vi "mailRapportExped.vi"(0 "chaine valves":string="12-216C-04521 EQIFIL 417mA 14.4ohm\t112105740008030109\t18.04.2008 15:35\tMQI\t12345/06-03.03.03\t2\t30\r\n12-216C-04521 EQIFIL 417mA 14.4ohm\t112105740008030108\t18.04.2008 15:35\tMQI\t12345/06-03.03.03\t2\t30\r\n12-216C-04521 EQIFIL 417mA 14.4ohm\t112105740008030107\t18.04.2008 15:35\tMQI\t12345/06-03.03.03\t2\t30\r\n12-216C-04521 EQIFIL 417mA 14.4ohm\t112105740008030106\t18.04.2008 15:35\tMQI\t12345/06-03.03.03\t2\t30\r\n12-216C-04521 EQIFIL 417mA 14.4ohm\t112105740008030105\t18.04.2008 15:35\tMQI\t12345/06-03.03.03\t2\t30\r\n12-216C-04521 EQIFIL 417mA 14.4ohm\t112105740008030104\t18.04.2008 15:35\tMQI\t12345/06-03.03.03\t1\t30\r\n12-216C-04521 EQIFIL 417mA 14.4ohm\t112105740008030103\t18.04.2008 15:34\tMQI\t12345/06-03.03.03\t1\t30\r\n12-216C-04521 EQIFIL 417mA 14.4ohm\t112105740008030102\t18.04.2008 15:34\tMQI\t12345/06-03.03.03\t1\t30\r\n12-216C-04521 EQIFIL 417mA 14.4ohm\t112105740008030101\t18.04.2008 15:34\tMQI\t12345/06-03.03.03\t1\t30\r\n12-216C-04521 EQIFIL 417mA 14.4ohm\t112105740008030100\t18.04.2008 15:34\tMQI\t12345/06-03.03.03\t1\t30\r\n12-216C-04521 EQIFIL 417mA 14.4ohm\t112105740008020106\t18.04.2008 15:34\tMQI\t12345/06-03.03.03\t1\t30\r\n12-216C-04521 EQIFIL 417mA 14.4ohm\t112105740008020105\t18.04.2008 15:34\tMQI\t12345/06-03.03.03\t1\t30\r\n12-216C-04521 EQIFIL 417mA 14.4ohm\t112105740008020104\t18.04.2008 15:34\tMQI\t12345/06-03.03.03\t1\t30\r\n12-216C-04521 EQIFIL 417mA 14.4ohm\t112105740008020103\t18.04.2008 15:34\tMQI\t12345/06-03.03.03\t1\t30\r\n12-216C-04521 EQIFIL 417mA 14.4ohm\t112105740008020102\t18.04.2008 15:34\tMQI\t12345/06-03.03.03\t1\t30\r\n12-216C-04521 EQIFIL 417mA 14.4ohm\t112105740008020101\t18.04.2008 15:34\tMQI\t12345/06-03.03.03\t1\t30\r\n12-216C-04521 EQIFIL 417mA 14.4ohm\t112105740008020100\t18.04.2008 15:34\tMQI\t12345/06-03.03.03\t1\t30\r\n12-216C-04521 EQIFIL 417mA 14.4ohm\t112105740008010112\t18.04.2008 15:34\tMQI\t12345/06-03.03.03\t1\t30\r\n12-216C-04521 EQIFIL 417mA 14.4ohm\t112105740008010111\t18.04.2008 15:34\tMQI\t12345/06-03.03.03\t1\t30\r\n12-216C-04521 EQIFIL 417mA 14.4ohm\t112105740008010110\t18.04.2008 15:34\tMQI\t12345/06-03.03.03\t1\t30\r\n12-216C-04521 EQIFIL 417mA 14.4ohm\t112105740008010109\t18.04.2008 15:34\tMQI\t12345/06-03.03.03\t1\t30\r\n12-216C-04521 EQIFIL 417mA 14.4ohm\t112105740008010108\t18.04.2008 15:34\tMQI\t12345/06-03.03.03\t1\t30\r\n12-216C-04521 EQIFIL 417mA 14.4ohm\t112105740008010107\t18.04.2008 15:34\tMQI\t12345/06-03.03.03\t1\t30\r\n12-216C-04521 EQIFIL 417mA 14.4ohm\t112105740008010106\t18.04.2008 15:34\tMQI\t12345/06-03.03.03\t1\t30\r\n12-216C-04521 EQIFIL 417mA 14.4ohm\t112105740008010105\t18.04.2008 15:34\tMQI\t12345/06-03.03.03\t1\t30\r\n12-216C-04521 EQIFIL 417mA 14.4ohm\t112105740008010104\t18.04.2008 15:34\tMQI\t12345/06-03.03.03\t1\t30\r\n12-216C-04521 EQIFIL 417mA 14.4ohm\t112105740008010103\t18.04.2008 15:33\tMQI\t12345/06-03.03.03\t1\t30\r\n12-216C-04521 EQIFIL 417mA 14.4ohm\t112105740008010102\t18.04.2008 15:33\tMQI\t12345/06-03.03.03\t1\t30\r\n12-216C-04521 EQIFIL 417mA 14.4ohm\t112105740008010101\t18.04.2008 15:33\tMQI\t12345/06-03.03.03\t1\t30\r\n12-216C-04521 EQIFIL 417mA 14.4ohm\t112105740008010100\t18.04.2008 15:33\tMQI\t12345/06-03.03.03\t1\t30\r\n", 3 "produit":string, 5 "DATA cmde":T1, 7 "chemin de base":path, 9 "Email Expédition":string="marion.quiquerez@fas.ch", 11 "error in (no error)":errorcluster caption="entrée d'erreur (pas d'erreur)", 12 "n° cmde":string, 14 "tab histo filtré\n par n° cmde":string[][](array[string])) -> (4 "Texte fichier":string, 6 "Titre fichier":string, 15 "error out":errorcluster caption="sortie d'erreur")   [LabVIEW 2020]
doc: "Envoi un mail avec la liste des valves emballées en pièce jointe si spécifié dans le fichier XML PP de la valve (FlatProp) ou correspondance produit code barre.txt (autres valves)"
uses:
  <vilib>/Utility/SMTP/NI_SMTPEmail.lvlib
panel:
  out "valeur max":string
  out "Texte mail":string caption="Résultat"
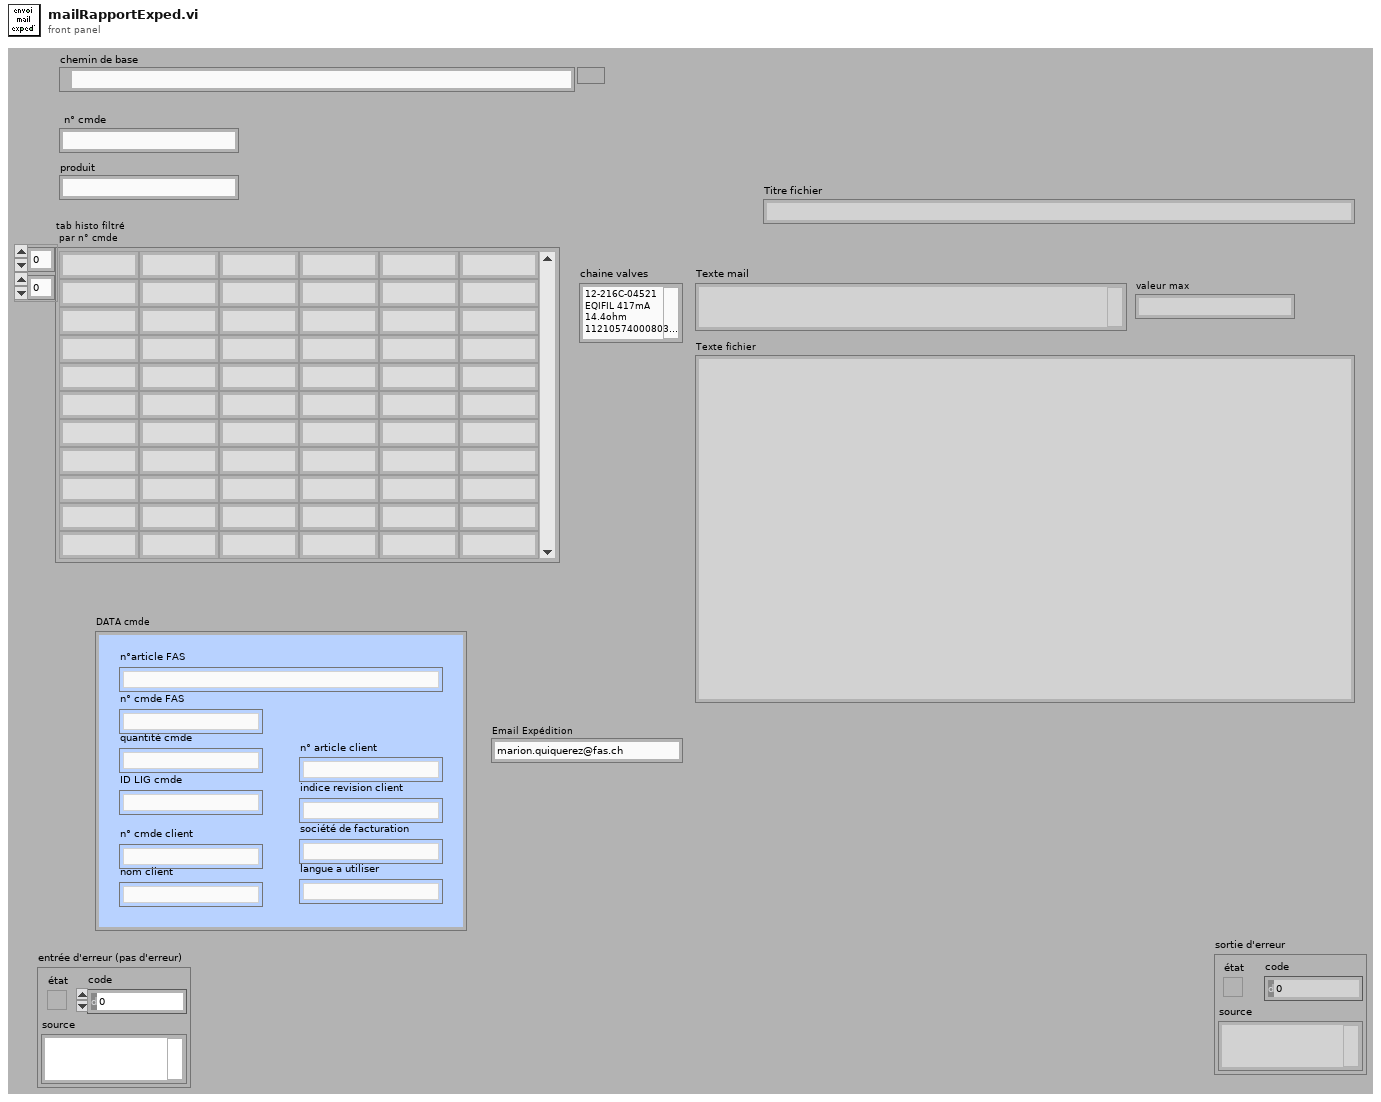
[diagram p1: front panel]
types:
  T1 = typedef "DATA commande.ctl" = cluster{"n°article FAS":string, "n° cmde FAS":string, "quantité cmde":string, "ID LIG cmde":string, "n° cmde client":string, "nom client":string, "n° article client":string, "indice revision client":string, "société de facturation":string, "langue a utiliser":string}
  T2 = enum16{"open", "replace", "create", "open or create", "replace or create", "replace or create with confirmation"}
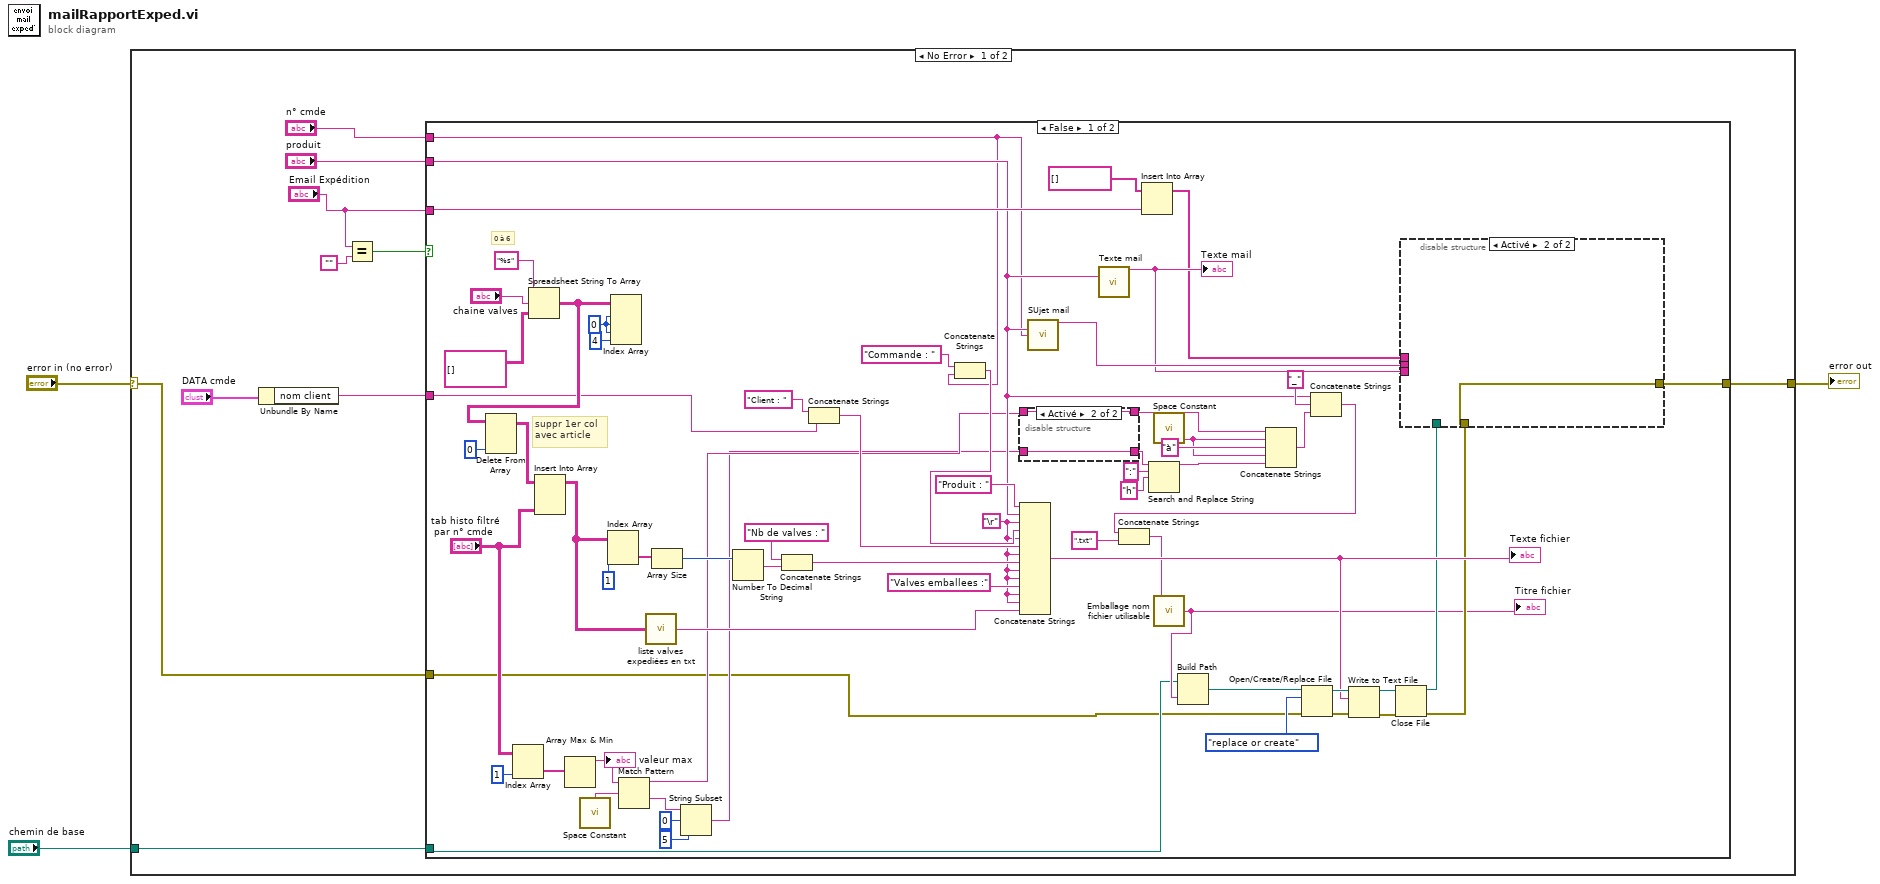
[diagram p0: block diagram]
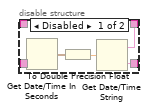
[diagram p2: hidden frame]
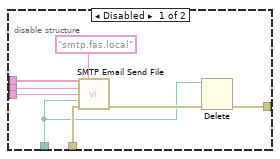
[diagram p3: hidden frame]
diagram:
  n1 = case shown="No Error" "error in (no error)" {
    selector: "error in (no error)" -> [w12 w96]
    tunnel: [w13 w96] -> w3
    tunnel: "chemin de base" -> [w4 _]
    frame No Error {
      n2 = Unbundle By Name("DATA cmde") -> ("nom client"=w7:string)
      n3 = Equal?(x="Email Expédition", y="") -> (x = y?=w9:bool)
      n4 = case shown="False" w9 {
        tunnel: [w53 w95] -> w13
        tunnel: w12 -> [w14 w95]
        tunnel: "Email Expédition" -> [w30 _]
        tunnel: w7 -> [w32 _]
        tunnel: "produit" -> [w27 _]
        tunnel: "n° cmde" -> [w26 _]
        tunnel: w4 -> [w15 _]
        frame False {
          w62 = 0 ("indice désactivé (col)")
          w49 = "\r"
          # "suppr 1er col \navec article"
          # "0 à 6"
          n5 = Index Array(array="tab histo filtré\n par n° cmde", index (col)=1 ("indice désactivé (col)")) -> (element=w23:string[])  [unwired: 1 in]
          n6 = Spreadsheet String To Array(format string="%s" ("chaîne de format"), spreadsheet string="chaine valves", array type (2D Dbl)=string[][] [] ("type de tableau (2D de dbl)")) -> (array=w36:string[][])  [unwired: 1 in]
          n7 = Delete From Array(array=w36, index (col)=0 ("indice désactivé (col)")) -> (array with subset deleted=w34:string[][])  [unwired: 2 in, 1 out]
          n8 = Insert Into Array(array=w34, new element="tab histo filtré\n par n° cmde") -> (w31:string[][])  [unwired: 2 in]
          n9 = Array Max & Min(array=w23) -> (max value=w22:string)  [unwired: 3 out]
          "valeur max" <- w22
          n10 = call <vilib>:"Space Constant.vi"() -> ("String"=w21:string)
          n11 = Index Array(array=w31, index (col)=1 ("indice désactivé (col)")) -> (element=w58:string[])  [unwired: 1 in]
          n12 = Index Array(array=w36, index (row) #1=w62, index (col) #1=w62, index (row) #2=w62, index (col) #2=4 ("indice désactivé (col)")) -> ()  [unwired: 2 out]
          n13 = Match Pattern(string=w22, regular expression=w21) -> (before substring=w20:string, after substring=w19:string)  [unwired: 1 in, 2 out]
          n14 = call "liste valves expediées en txt.vi"("Tab valves"=w31) -> ("liste valves"=w50:string)
          n15 = Array Size(array=w58) -> (size(s)=w33:i32)
          n16 = String Subset(string=w19, offset (0)=0, length (rest)=5 ("longueur (reste)")) -> (substring=w16:string)
          n17 = Number To Decimal String(number=w33) -> (decimal integer string=w56:string)  [unwired: 1 in]
          n18 = Concatenate Strings("Nb de valves : " ("expression régulière"), w56) -> (w73:string)
          n19 = Concatenate Strings("Client : " ("expression régulière"), w32) -> (w51:string)
          n20 = Concatenate Strings("Commande : " ("expression régulière"), w26) -> (w74:string)
          n21 = disable-structure shown="Activé" {
            disable-tunnel: [w81 w84] -> w42
            disable-tunnel: [w80 w85] -> w39
            disable-tunnel: w20 -> [_ w85]
            disable-tunnel: w16 -> [_ w84]
            frame Disabled {
              n22 = Get Date/Time In Seconds() -> (seconds since 1Jan1904=w82:timestamp)
              n23 = To Double Precision Float(number=w82) -> (double precision float=w83:dbl)
              n24 = Get Date/Time String(seconds (now)=w83) -> (date string=w80:string, time string=w81:string)  [unwired: 2 in]
            }
            frame Enabled {
            }
          }
          n25 = Concatenate Strings("Produit : " ("expression régulière"), w27, w49, w74, w49, w51, w49, w73, w49, w49, "Valves emballees :" ("chaîne"), w49, w49, w50) -> (w69:string)
          "Texte fichier" <- w69
          n26 = call "SUjet mail"("produit"=w27, "n° cmde"=w26) -> ("Result"=w79:string)  [unwired: 12 in, 1 out]
          n27 = call "Texte mail"("produit"=w27) -> ("Result"=w78:string)  [unwired: 13 in, 1 out]
          "Texte mail" <- w78
          n28 = Insert Into Array(array=string[] [] ("recipients"), new element=w30) -> (w76:string[])  [unwired: 1 in]
          n29 = Search and Replace String(input string=w42, search string=":" ("chaîne recherchée"), replace string="h" ("chaîne de remplacement (\"\")")) -> (result string=w40:string)  [unwired: 5 in, 3 out]
          n30 = call <vilib>:"Space Constant.vi"() -> ("String"=w38:string)
          n31 = Concatenate Strings(w39, w38, "à" ("chaîne"), w38, w40) -> (w37:string)
          n32 = Concatenate Strings(w27, "_", w37) -> (w47:string)
          n33 = Concatenate Strings(w47, ".txt" ("chaîne")) -> (w29:string)
          n34 = call "Emballage nom fichier utilisable.vi"("chaîne en entrée"=w29) -> ("chaîne résultante"=w28:string)
          "Titre fichier" <- w28
          n35 = Build Path(base path=w15, name or relative path=w28) -> (appended path=w46:path)
          n36 = Open/Create/Replace File(file path (use dialog)=w46, error in=w14, operation (0:open)=T2."replace or create" ("opération (0 : open)")) -> (refnum out=w70:refnum<file>, error out=w72:errorcluster)  [unwired: 3 in, 1 out]
          n37 = Write to Text File(file (use dialog)=w70, text=w69, error in=w72) -> (refnum out=w67:refnum<file>, error out=w68:errorcluster)  [unwired: 1 in, 1 out]
          n38 = Close File(refnum=w67, error in=w68) -> (path=w48:path, error out=w66:errorcluster)
          n39 = disable-structure shown="Activé" {
            disable-tunnel: w79 -> [w92 _]
            disable-tunnel: w78 -> [w91 _]
            disable-tunnel: w76 -> [w90 _]
            disable-tunnel: w66 -> [w89 w94]
            disable-tunnel: [w87 w94] -> w53
            disable-tunnel: w48 -> [w86 _]
            frame Disabled {
              n40 = call <vilib>:"SMTP Email Send File.vi"("recipients"=w90, "mail server"="smtp.fas.local", "subject ([No Subject])"=w92, "message"=w91, "file path"=w86, "error in (no error)"=w89) -> ("error out"=w88:errorcluster)  [unwired: 8 in, 1 out]
              n41 = Delete(path (use dialog)=w86, error in=w88) -> (error out=w87:errorcluster)  [unwired: 3 in, 2 out]
            }
            frame Enabled {
            }
          }
        }
        frame True {
        }
      }
    }
    frame Error {
    }
  }
  "error out" <- w3
